vi "IRF Tail Analysis.vi"(8 "error in (no error)":errorcluster, 11 "Plot in":cluster{"t Array":dbl[], "Array":dbl[]}) -> (0 "error out":errorcluster, 1 "Tail Sum":dbl, 2 "Tail Start":dbl, 3 "Plot out":cluster{"t Array":dbl[], "Array":dbl[]}, 4 "Tail Min":dbl)   [LabVIEW 2021, in "Fits.lvlib"]
uses:
  Fits.lvlib
  26090ace-848f-4d15-9d49-f1162b1a5ca8.vi
panel:
  # "see the License on the block diagram (Ctrl+E or Window:Show Block Diagram)"
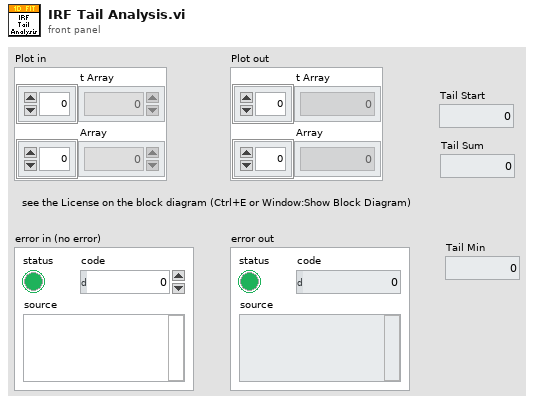
[diagram p1: front panel]
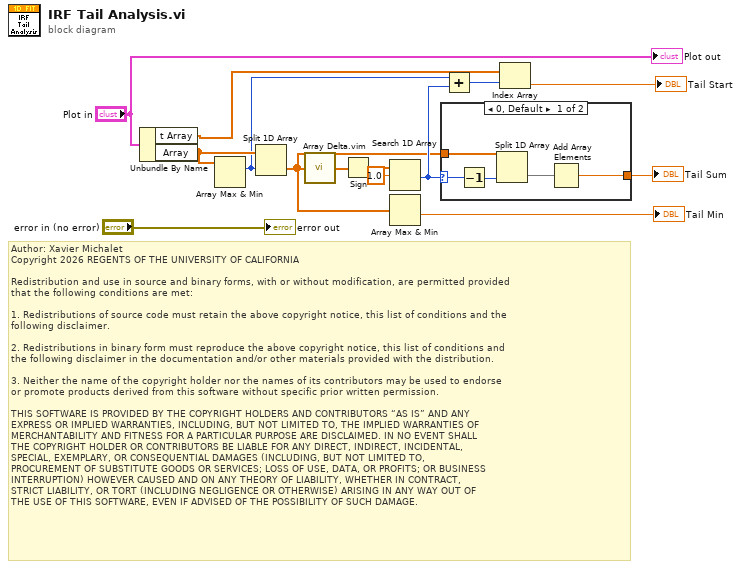
[diagram p0: block diagram]
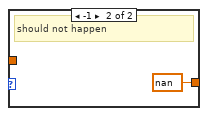
[diagram p2: hidden frame]
diagram:
  # "Author: Xavier Michalet\nCopyright 2026 REGENTS OF THE UNIVERSITY OF CALIFORNIA\n\nRedistribution and use in source and binary forms, with or without modification, are permitted provided\nthat the following conditions are met:\n\n1. Redistributions of source code must retain the above copyright notice, this list of conditions and the\nfollowing disclaimer.\n\n2. Redistributions in binary form must reproduce the above copyright notice, this list of conditions and\nthe following disclaimer in the documentation and/or other materials provided with the distribution.\n\n3. Neither the name of the copyright holder nor the names of its contributors may be used to endorse \nor promote products derived from this software without specific prior written permission.\n\nTHIS SOFTWARE IS PROVIDED BY THE COPYRIGHT HOLDERS AND CONTRIBUTORS “AS IS” AND ANY \nEXPRESS OR IMPLIED WARRANTIES, INCLUDING, BUT NOT LIMITED TO, THE IMPLIED WARRANTIES OF\nMERCHANTABILITY AND FITNESS FOR A PARTICULAR PURPOSE ARE DISCLAIMED. IN NO EVENT SHALL\nTHE COPYRIGHT HOLDER OR CONTRIBUTORS BE LIABLE FOR ANY DIRECT, INDIRECT, INCIDENTAL, \nSPECIAL, EXEMPLARY, OR CONSEQUENTIAL DAMAGES (INCLUDING, BUT NOT LIMITED TO, \nPROCUREMENT OF SUBSTITUTE GOODS OR SERVICES; LOSS OF USE, DATA, OR PROFITS; OR BUSINESS\nINTERRUPTION) HOWEVER CAUSED AND ON ANY THEORY OF LIABILITY, WHETHER IN CONTRACT, \nSTRICT LIABILITY, OR TORT (INCLUDING NEGLIGENCE OR OTHERWISE) ARISING IN ANY WAY OUT OF\nTHE USE OF THIS SOFTWARE, EVEN IF ADVISED OF THE POSSIBILITY OF SUCH DAMAGE."
  n1 = Unbundle By Name("Plot in") -> ("t Array"=w4:dbl[], "Array"=w12:dbl[])
  n2 = Array Max & Min(array=w12) -> (max index (indices)=w7:i32)  [unwired: 3 out]
  n3 = Split 1D Array(array=w12, index=w7) -> (second subarray=w2:dbl[])  [unwired: 1 out]
  n4 = call "Array Delta.vim"("A"=w2) -> ("A[i+1]-A[i]"=w11:dbl[])  [unwired: 8 in]
  n5 = Sign(1:w11) -> (0:w10:dbl[])
  n6 = Search 1D Array(1D array=w10, element=1.0) -> (index of element=w6:i32)  [unwired: 1 in]
  n7 = Array Max & Min(array=w2) -> (min value=→"Tail Min":dbl)  [unwired: 3 out]
  n8 = case shown="0, Default" w6 {
    selector: w6 -> [w19 _]
    tunnel: w2 -> [w17 _]
    tunnel: [w15 nan ("Numeric")] -> w8
    frame 0, Default {
      n9 = Decrement(x=w19) -> (x-1=w18:i32)
      n10 = Split 1D Array(array=w17, index=w18) -> (second subarray=w16:dbl[])  [unwired: 1 out]
      n11 = Add Array Elements(numeric array=w16) -> (sum=w15:dbl)
    }
    frame -1 {
      # "should not happen"
    }
  }
  "Tail Sum" <- w8
  n12 = Add(x=w7, y=w6) -> (x+y=w5:i32)
  n13 = Index Array(array=w4, index=w5) -> (element=→"Tail Start":dbl)
  "error out" <- "error in (no error)"
  "Plot out" <- "Plot in"
